vi "NumIntegrate_Rkdp_Func_B1B2.vi"(11 "Index":i32) -> (3 "RKDP_B1-B2":dbl)   [LabVIEW 2019, in "Trajectory_Library.lvlib"]
doc: "Internal function used by Rkdp_Impl.vi\n\nInputs:\n - Index -- Index into B1 and B2 array (must be 0 - 6 )\n\nOutputs:\n - B1B2 -- Value of B1 - B2 looked up by index."
uses:
  Trajectory_Library.lvlib
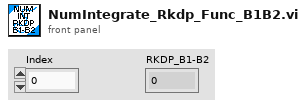
[diagram p1: front panel]
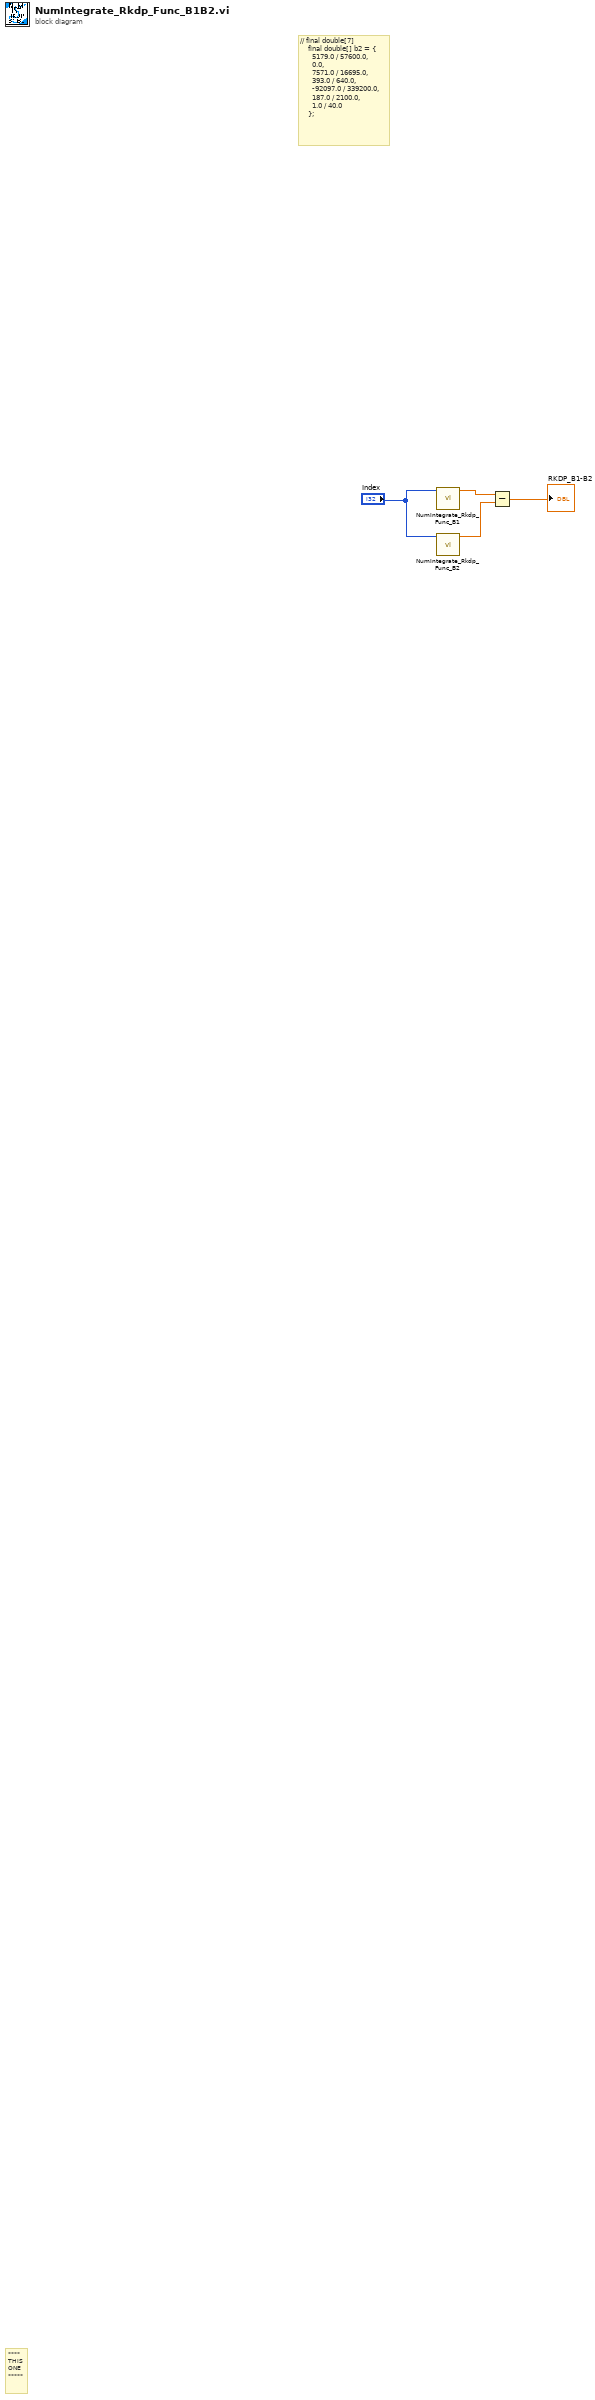
[diagram p0: block diagram]
diagram:
  # "// final double[7]\n    final double[] b2 = {\n      5179.0 / 57600.0,\n      0.0,\n      7571.0 / 16695.0,\n      393.0 / 640.0,\n      -92097.0 / 339200.0,\n      187.0 / 2100.0,\n      1.0 / 40.0\n    };"
  # "****\nTHIS\nONE\n*****"
  n1 = call "NumIntegrate_Rkdp_Func_B1.vi"("Index"="Index") -> ("RKDP_B1"=w4:dbl)  [unwired: 10 in]
  n2 = call "NumIntegrate_Rkdp_Func_B2.vi"("Index"="Index") -> ("RKDP_B2"=w3:dbl)  [unwired: 10 in]
  n3 = Subtract(x=w4, y=w3) -> (x-y=→"RKDP_B1-B2":dbl)
